vi "Do.vi"(8 "error in (no error)":errorcluster, 10 "Actor in":refnum<class "Actor.lvclass">, 11 "update nested DVR on caller Msg":refnum<class "update nested DVR on caller Msg.lvclass">) -> (0 "error out":errorcluster, 2 "Actor out":refnum<class "Actor.lvclass">)   [LabVIEW 2020, in "Template.lvlib" / "update nested DVR on caller Msg.lvclass"]
doc: "This VI delivers the message to the actor by calling the appropriate method(s) on the actor."
uses:
  update nested DVR on caller Msg.lvclass
  <vilib>/ActorFramework/Actor/Actor.lvclass
  template/Template.lvclass
  C:/Program Files/National Instruments/LabVIEW 2020/vi.lib/ActorFramework/Actor/Actor.lvclass
  9ef47adc-f318-494c-9b8b-6df3216d6863.vi
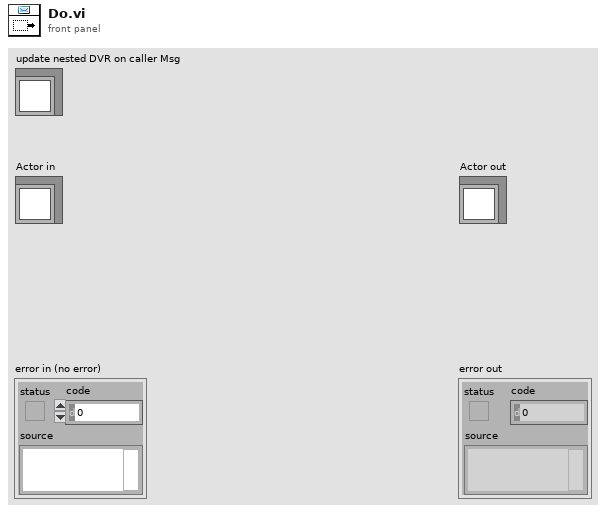
[diagram p1: front panel]
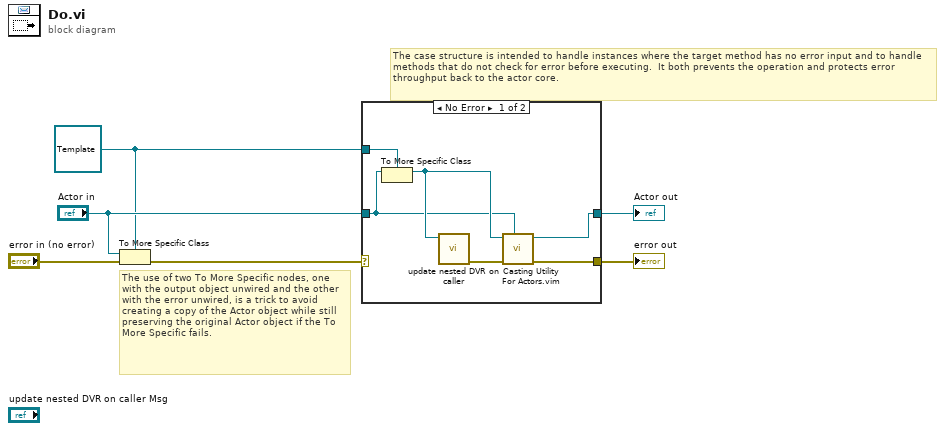
[diagram p0: block diagram]
diagram:
  w1 = refnum<class "Template.lvclass"> refnum ("Actor in")
  # "The use of two To More Specific nodes, one with the output object unwired and the other with the error unwired, is a trick to avoid creating a copy of the Actor object while still preserving the original Actor object if the To More Specific fails."
  # "The case structure is intended to handle instances where the target method has no error input and to handle methods that do not check for error before executing.  It both prevents the operation and protects error throughput back to the actor core."
  n1 = To More Specific Class(target class=w1, reference="Actor in", error in="error in (no error)") -> (error out=w5:errorcluster)  [unwired: 1 out]
  n2 = case shown="No Error" w5 {
    selector: w5 -> [_ w14]
    tunnel: [w8 w14] -> w4
    tunnel: [w9 w13] -> w3
    tunnel: "Actor in" -> [w10 w13]
    tunnel: w1 -> [w11 _]
    frame No Error {
      n3 = To More Specific Class(target class=w11, reference=w10) -> (specific class reference=w12:refnum<class "Template.lvclass">)  [unwired: 1 in, 1 out]
      n4 = call "update nested DVR on caller.vi"("Template in"=w12) -> ("error out"=w7:errorcluster)  [unwired: 10 in]
      n5 = call "Casting Utility For Actors.vim"("type"=w10, "error in (no error)"=w7, "Actor in"=w12) -> ("error out"=w8:errorcluster, "Actor out"=w9:refnum<class "Actor.lvclass">)  [unwired: 7 in]
    }
    frame Error {
      # "If type check fails, pass the original object out again."
    }
  }
  "error out" <- w4
  "Actor out" <- w3
